vi "json reciebe.vi"() -> ()   [LabVIEW 2025]
uses:
  <vilib>/httpClient/LabVIEWHTTPClient.lvlib
panel:
  out "Rele":bool
  out "Hora":string
  out "Fecha":string
  out "Accionamiento":dbl
  in  "stop":bool
  out "error out":errorcluster
  out "body":string
  out "headers":string
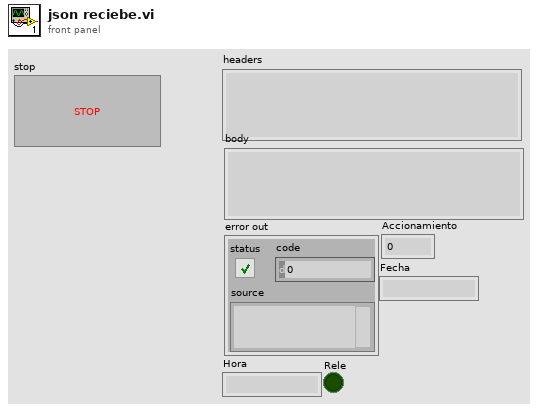
[diagram p1: front panel]
types:
  T1 = cluster{"Accionamiento":dbl, "Fecha":string, "Hora":string, "Rele":bool}
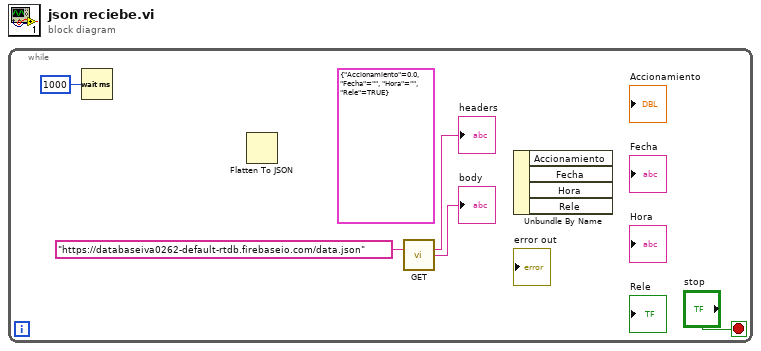
[diagram p0: block diagram]
diagram:
  n1 = while {
    stop <- "stop" stop-if-true
    (unwired) T1 {"Accionamiento"=0.0, "Fecha"="", "Hora"="", "Rele"=TRUE}
    n2 = Wait (ms)(milliseconds to wait=u32 1000) -> ()  [unwired: 1 out]
    n3 = Flatten To JSON() -> ()  [unwired: 3 in, 2 out]
    n4 = call <vilib>:"GET.vi"("url"="https://databaseiva0262-default-rtdb.firebaseio.com/data.json") -> ("headers"=→"headers":string, "body"=→"body":string)  [unwired: 11 in, 2 out]
    n5 = Unbundle By Name() -> ()  [unwired: 1 in, 4 out]
  }
